vi "NMRController.vi"() -> ()   [LabVIEW 2023]
uses:
  typeDefs/TimeUnits.ctl
  typeDefs/SystemStates.ctl
  <vilib>/DAQmx/write.llb/DAQmx Write (Analog 1D DBL 1Chan NSamp).vi
  <vilib>/DAQmx/read.llb/DAQmx Read (Analog DBL 1Chan 1Samp).vi
  <vilib>/DAQmx/create/channels.llb/DAQmx Create Channel (AI-Voltage-Basic).vi
  <vilib>/DAQmx/configure/timing.llb/DAQmx Timing (Sample Clock).vi
  <vilib>/DAQmx/configure/trigger.llb/DAQmx Start Trigger (Digital Edge).vi
  <vilib>/DAQmx/create/channels.llb/DAQmx Create Channel (AO-Voltage-Basic).vi
  <vilib>/DAQmx/miscellaneous.llb/DAQmx Fill In Error Info.vi
panel:
  in  "STOP":bool
  in  "NMR Signal":tag
  in  "Calibration Antenna":tag
  in  "External Start":tag
  in  "Timed Trigger":bool
  in  "Trigger":bool
  in  "Time Units":T1
  in  "Gathering Time":dbl
  in  "Settings":bool
  out "Voltage Data":dbl[](graph)
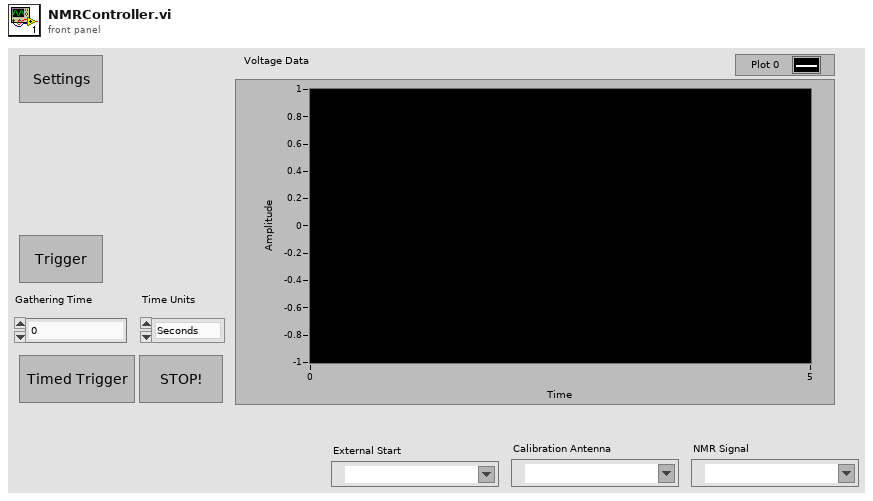
[diagram p1: front panel]
types:
  T1 = typedef "TimeUnits.ctl" = enum16{"Seconds", "Minutes", "Hours"}
  T2 = typedef "SystemStates.ctl" = enum16{"Idle", "Initialize", "Acquire", "Stop", "Shutdown", "Calibrate", "Settings", "I/O"}
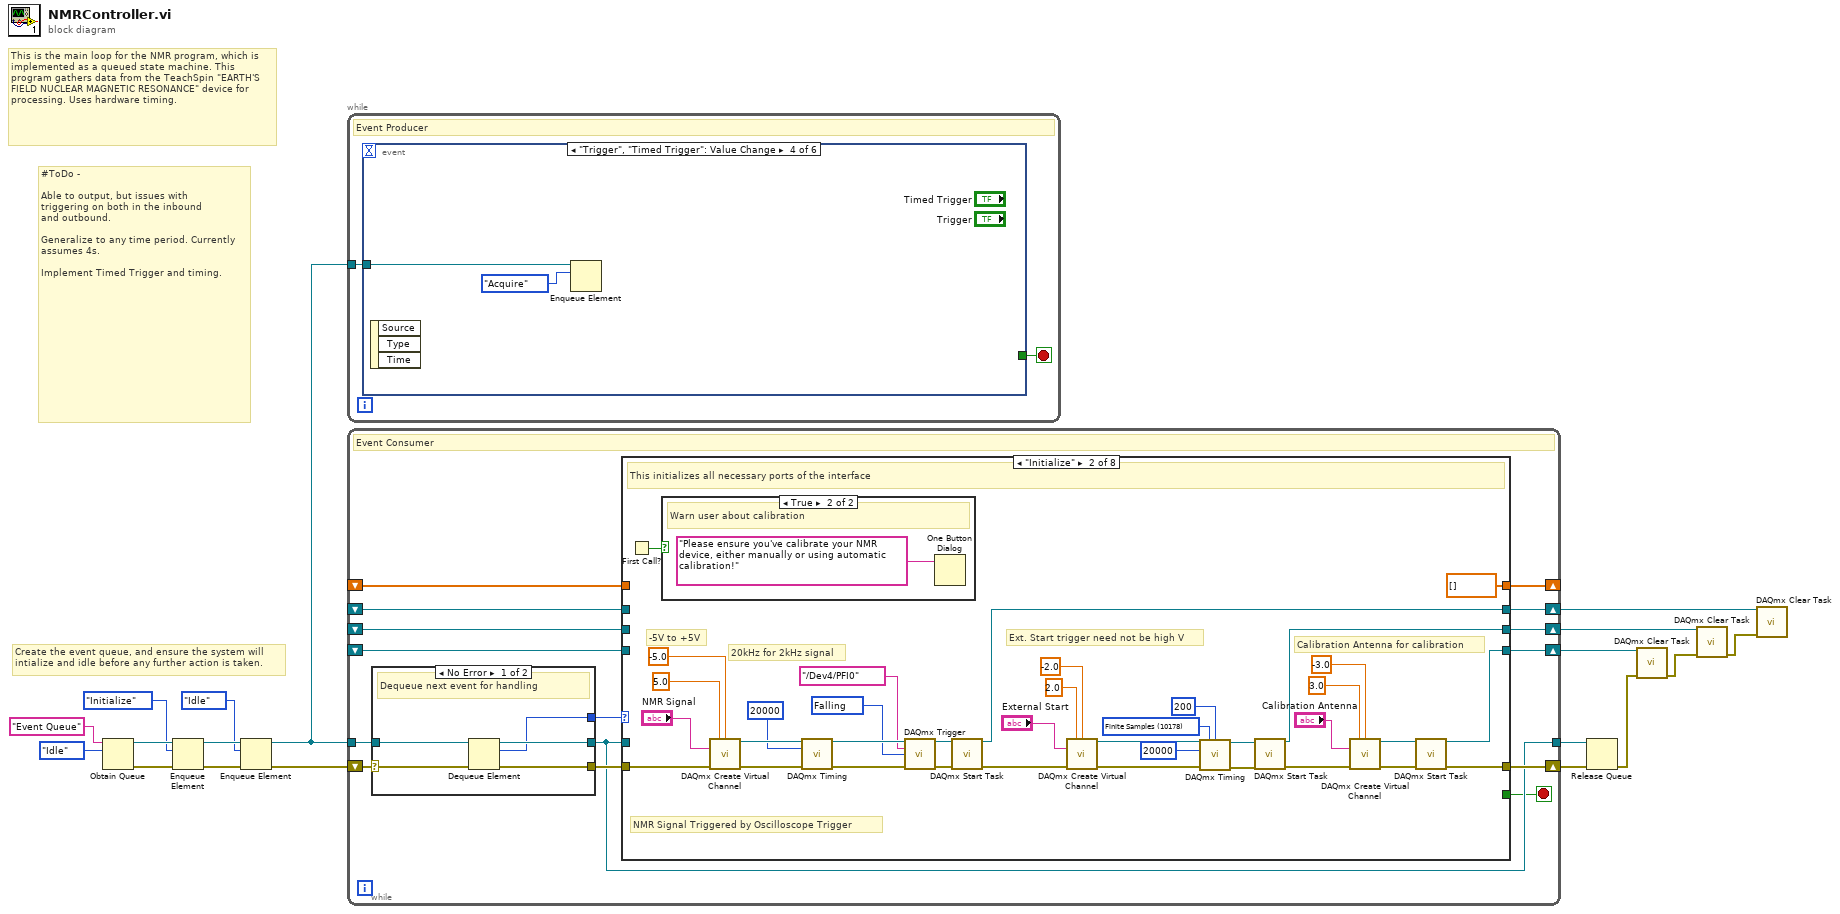
[diagram p0: block diagram]
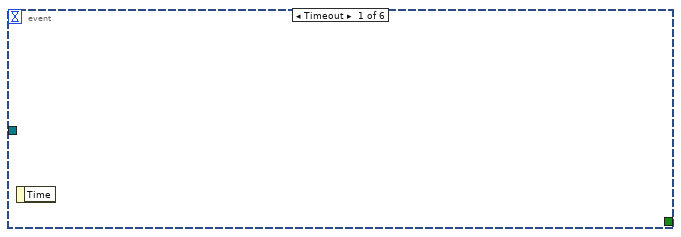
[diagram p2: hidden frame]
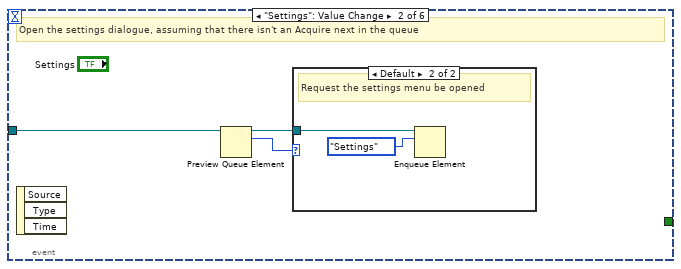
[diagram p3: hidden frame]
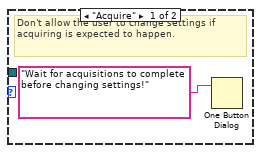
[diagram p4: hidden frame]
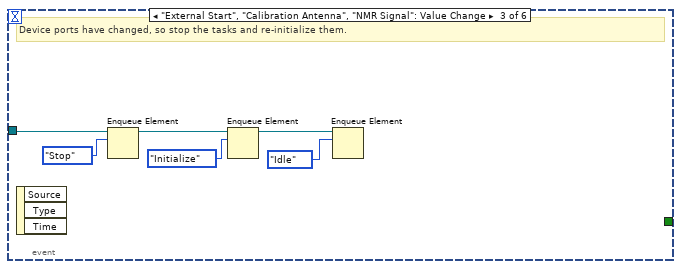
[diagram p5: hidden frame]
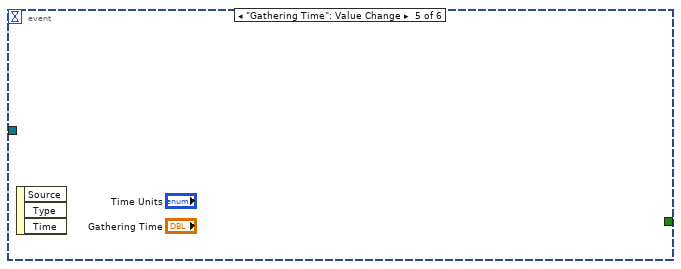
[diagram p6: hidden frame]
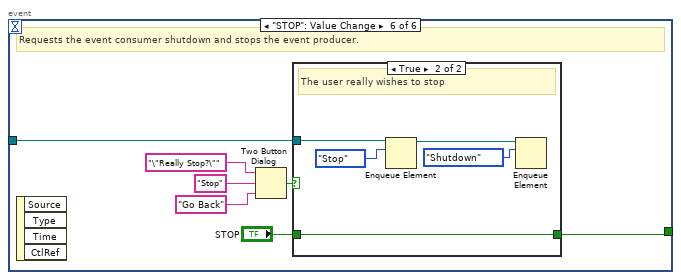
[diagram p7: hidden frame]
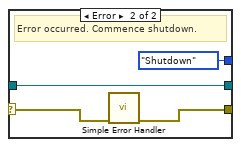
[diagram p9: hidden frame]
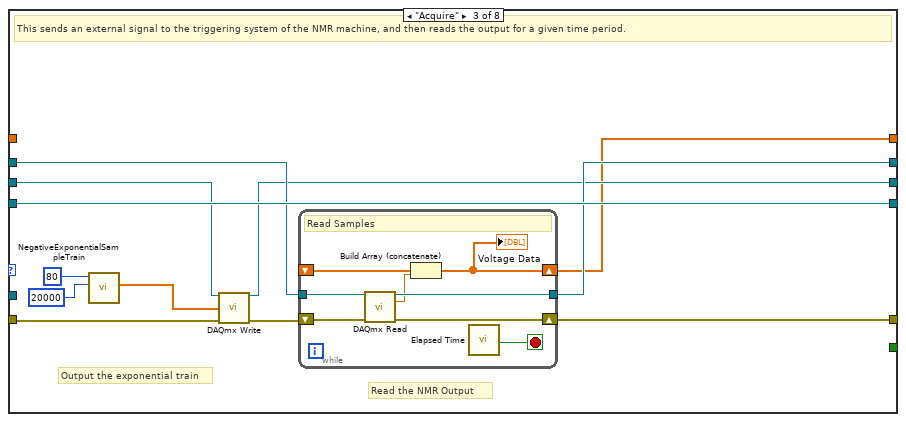
[diagram p12: hidden frame]
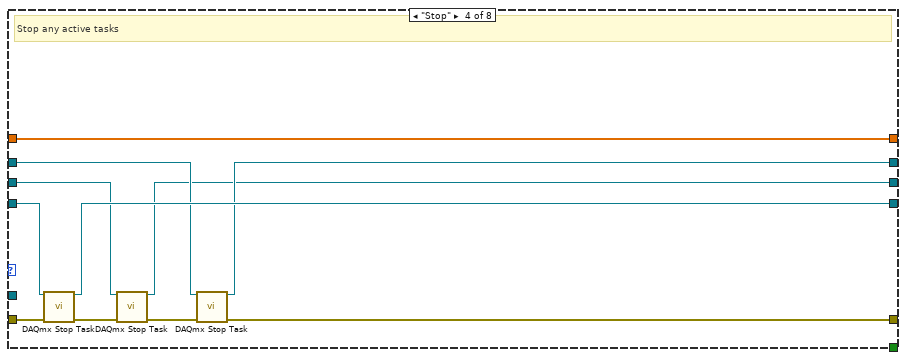
[diagram p13: hidden frame]
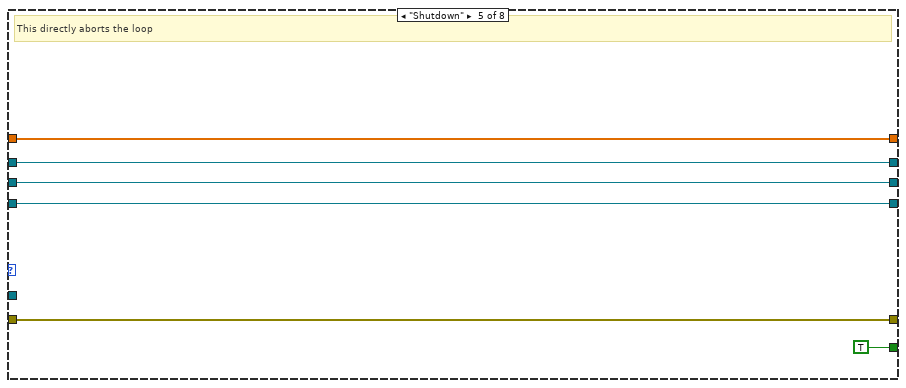
[diagram p14: hidden frame]
diagram:
  # "#ToDo - \n\nAble to output, but issues with\ntriggering on both in the inbound\nand outbound.\n\nGeneralize to any time period. Currently assumes 4s.\n\nImplement Timed Trigger and timing."
  # "This is the main loop for the NMR program, which is implemented as a queued state machine. This program gathers data from the TeachSpin \"EARTH'S FIELD NUCLEAR MAGNETIC RESONANCE\" device for processing. Uses hardware timing."
  # "Create the event queue, and ensure the system will intialize and idle before any further action is taken."
  n1 = Obtain Queue(name (unnamed)="Event Queue", element data type=SystemStates."Idle" ("States")) -> (queue out=w17:refnum<queue>, error out=w13:errorcluster)  [unwired: 3 in, 1 out]
  n2 = Enqueue Element(queue=w17, element=SystemStates."Initialize", error in (no error)=w13) -> (queue out=w16:refnum<queue>, error out=w12:errorcluster)  [unwired: 1 in, 1 out]
  n3 = Enqueue Element(queue=w16, element=SystemStates."Idle", error in (no error)=w12) -> (queue out=w15:refnum<queue>, error out=w14:errorcluster)  [unwired: 1 in, 1 out]
  n4 = while {
    tunnel: w15 -> [w20]
    stop <- w19 stop-if-true
    # "Event Producer"
    n5 = event shown="[3] \"Trigger\", \"Timed Trigger\": Value Change" {
      selector: _ -> [_ _ _ _ _ _]
      dyn-events: _ -> [_ _ _ _ _ _]
      timeout: _ -> [_ _ _ _ _ _]
      tunnel: w20 -> [_ w23 w32 w34 _ w38]
      tunnel: [_ _ _ _ _ w35] -> w19
      event Timeout {
        n6 = event-data() -> ()  [unwired: 1 in, 1 out]
      }
      event "Settings": Value Change {
        # "Open the settings dialogue, assuming that there isn't an Acquire next in the queue"
        n7 = event-data() -> ()  [unwired: 1 in, 3 out]
        n8 = Preview Queue Element(queue=w23) -> (queue out=w21:refnum<queue>, element=w22:T2)  [unwired: 2 in, 2 out]
        n9 = case shown="Default" w22 {
          tunnel: w21 -> [_ w25]
          frame "Acquire" {
            # "Don't allow the user to change settings if acquiring is expected to happen."
            n10 = One Button Dialog(message="Wait for acquisitions to complete before changing settings!") -> ()  [unwired: 1 in, 1 out]
          }
          frame Default {
            # "Request the settings menu be opened"
            n11 = Enqueue Element(queue=w25, element=SystemStates."Settings") -> ()  [unwired: 2 in, 3 out]
          }
        }
      }
      event "External Start", "Calibration Antenna", "NMR Signal": Value Change {
        # "Device ports have changed, so stop the tasks and re-initialize them."
        n12 = event-data() -> ()  [unwired: 1 in, 3 out]
        n13 = Enqueue Element(queue=w32, element=SystemStates."Stop") -> (queue out=w30:refnum<queue>)  [unwired: 2 in, 2 out]
        n14 = Enqueue Element(queue=w30, element=SystemStates."Initialize") -> (queue out=w29:refnum<queue>)  [unwired: 2 in, 2 out]
        n15 = Enqueue Element(queue=w29, element=SystemStates."Idle") -> ()  [unwired: 2 in, 3 out]
      }
      event "Trigger", "Timed Trigger": Value Change {
        n16 = event-data() -> ()  [unwired: 1 in, 3 out]
        n17 = Enqueue Element(queue=w34, element=SystemStates."Acquire") -> ()  [unwired: 2 in, 3 out]
      }
      event "Gathering Time": Value Change {
        n18 = event-data() -> ()  [unwired: 1 in, 3 out]
      }
      event "STOP": Value Change {
        # "Requests the event consumer shutdown and stops the event producer."
        n19 = event-data() -> ()  [unwired: 1 in, 4 out]
        n20 = Two Button Dialog(message="\"Really Stop?\"", 1:"Go Back" ("F button name (\"Cancel\")"), 2:"Stop" ("T button name (\"OK\")")) -> (T button?=w37:bool)
        n21 = case shown="True" w37 {
          tunnel: w38 -> [_ w43]
          tunnel: "STOP" -> [_ w42]
          tunnel: [_ w42] -> w35
          frame False {
            # "The user wants to go back"
          }
          frame True {
            # "The user really wishes to stop"
            n22 = Enqueue Element(queue=w43, element=SystemStates."Stop") -> (queue out=w45:refnum<queue>)  [unwired: 2 in, 2 out]
            n23 = Enqueue Element(queue=w45, element=SystemStates."Shutdown") -> ()  [unwired: 2 in, 3 out]
          }
        }
      }
    }
  }
  n24 = while {
    tunnel: w15 -> [w58]
    shift-right: [w61] -> w7
    shift-left: w14 -> [w59]
    tunnel: [w55] -> w8
    shift-right: [w56] -> w6
    shift-left: _ -> [w53]
    shift-right: [w52] -> w4
    shift-left: _ -> [w51]
    shift-right: [w50] -> w3
    shift-left: _ -> [w49]
    shift-right: [w48] -> _
    shift-left: _ -> [w47]
    stop <- w54 stop-if-true
    # "Event Consumer"
    n25 = case shown="No Error" w59 {
      selector: w59 -> [w66 w68]
      tunnel: [w65 w67] -> w60
      tunnel: w58 -> [w64 w69]
      tunnel: [w63 w69] -> w55
      tunnel: [w62 SystemStates."Shutdown" ("States")] -> w57
      frame No Error {
        # "Dequeue next event for handling"
        n26 = Dequeue Element(queue=w64, error in (no error)=w66) -> (queue out=w63:refnum<queue>, element=w62:T2, error out=w65:errorcluster)  [unwired: 1 in, 1 out]
      }
      frame Error {
        # "Error occurred. Commence shutdown."
        n27 = call <vilib>:"Simple Error Handler.vi"("error in (no error)"=w68) -> ("error out"=w67:errorcluster)  [unwired: 4 in, 4 out]
      }
    }
    n28 = case shown="\"Initialize\"" w57 {
      tunnel: [w75 w91 w123 w141 w149 w154 w159 w164] -> w61
      tunnel: w60 -> [w75 w110 w119 w142 w149 w154 w159 w164]
      tunnel: w55 -> [_ _ _ _ _ _ _ _]
      tunnel: [w74 w90 w124 w140 w147 w153 w158 w163] -> w56
      tunnel: [_ _ _ _ TRUE _ _ _] -> w54
      tunnel: w53 -> [w74 _ w124 w143 w147 w153 w158 w163]
      tunnel: [w73 w98 w121 w138 w146 w152 w157 w162] -> w52
      tunnel: w51 -> [w73 _ w122 w139 w146 w152 w157 w162]
      tunnel: [w72 w88 w114 w134 w145 w151 w156 w161] -> w50
      tunnel: w49 -> [w72 _ w115 w135 w145 w151 w156 w161]
      tunnel: [w71 dbl[] [] w113 w133 w144 w150 w155 w160] -> w48
      tunnel: w47 -> [w71 _ _ w133 w144 w150 w155 w160]
      frame "Idle", Default {
      }
      frame "Initialize" {
        w77 = 10171 items=["Rising"=10280, "Falling"=10171] ("edge")
        w83 = 10178 items=["Finite Samples"=10178, "Continuous Samples"=10123, "Hardware Timed Single Point"=12522] ("sample mode")
        # "Calibration Antenna for calibration"
        # "Ext. Start trigger need not be high V"
        # "NMR Signal Triggered by Oscilloscope Trigger"
        # "-5V to +5V"
        # "20kHz for 2kHz signal"
        # "This initializes all necessary ports of the interface"
        n29 = First Call?() -> (First Call?: T/F=w111:bool)
        n30 = case shown="True" w111 {
          frame False {
            # "Re-initialization, no need to warn the user"
          }
          frame True {
            # "Warn user about calibration"
            n31 = One Button Dialog(message="Please ensure you've calibrate your NMR device, either manually or using automatic calibration!" ("button name (\"OK\")")) -> ()  [unwired: 1 in, 1 out]
          }
        }
        n32 = call-poly <vilib>:"DAQmx Create Virtual Channel.vi"("maximum value"=5.0, "minimum value"=-5.0, "physical channels"="NMR Signal", "error in"=w110) -> ("task out"=w102:refnum<k21>, "error out"=w104:errorcluster)  [unwired: 10 in]
        n33 = call-poly <vilib>:"DAQmx Timing.vi"("task/channels in"=w102, "rate"=20000, "error in"=w104) -> ("task out"=w101:refnum<k21>, "error out"=w103:errorcluster)  [unwired: 11 in]
        n34 = call-poly <vilib>:"DAQmx Trigger.vi"("task/channels in"=w101, "source"=tag "/Dev4/PFI0", "edge"=w77, "error in"=w103) -> ("task out"=w99:refnum<k21>, "error out"=w97:errorcluster)  [unwired: 10 in]
        n35 = call <vilib>:"DAQmx Start Task.vi"("task/channels in"=w99, "error in"=w97) -> ("task out"=w98:refnum<k21>, "error out"=w96:errorcluster)  [unwired: 12 in]
        n36 = call-poly <vilib>:"DAQmx Create Virtual Channel.vi"("maximum value"=2.0, "minimum value"=-2.0, "physical channels"="External Start", "error in"=w96) -> ("task out"=w87:refnum<k21>, "error out"=w86:errorcluster)  [unwired: 10 in]
        n37 = call-poly <vilib>:"DAQmx Timing.vi"("task/channels in"=w87, "sample mode"=w83, "samples per channel"=200, "rate"=20000, "error in"=w86) -> ("task out"=w84:refnum<k21>, "error out"=w85:errorcluster)  [unwired: 9 in]
        n38 = call <vilib>:"DAQmx Start Task.vi"("task/channels in"=w84, "error in"=w85) -> ("task out"=w88:refnum<k21>, "error out"=w93:errorcluster)  [unwired: 12 in]
        n39 = call-poly <vilib>:"DAQmx Create Virtual Channel.vi"("maximum value"=3.0, "minimum value"=-3.0, "physical channels"="Calibration Antenna", "error in"=w93) -> ("task out"=w89:refnum<k21>, "error out"=w92:errorcluster)  [unwired: 10 in]
        n40 = call <vilib>:"DAQmx Start Task.vi"("task/channels in"=w89, "error in"=w92) -> ("task out"=w90:refnum<k21>, "error out"=w91:errorcluster)  [unwired: 12 in]
      }
      frame "Acquire" {
        # "Read the NMR Output"
        # "Output the exponential train"
        # "This sends an external signal to the triggering system of the NMR machine, and then reads the output for a given time period."
        n41 = call "NegativeExponentialSampleTrain.vi"("Sample rate"=20000 ("rate"), "Time (ms)"=80) -> ("ImpulseTrain"=w118:dbl[])  [unwired: 9 in]
        n42 = call-poly <vilib>:"DAQmx Write.vi"("task/channels in"=w115, "data"=w118, "error in"=w119) -> ("task out"=w114:refnum<k21>, "error out"=w120:errorcluster)  [unwired: 10 in, 1 out]
        n43 = while {
          shift-right: [w131] -> w123
          shift-left: w120 -> [w132]
          tunnel: w122 -> [w130]
          tunnel: [w129] -> w121
          shift-right: [w125] -> w113
          shift-left: _ -> [w126]
          stop <- w128 stop-if-true
          # "Read Samples"
          n44 = call-poly <vilib>:"DAQmx Read.vi"("task/channels in"=w130, "error in"=w132) -> ("task out"=w129:refnum<k21>, "data"=w127:dbl, "error out"=w131:errorcluster)  [unwired: 11 in]
          n45 = Build Array (concatenate)(w126, w127) -> (w125:dbl[])
          "Voltage Data" <- w125
          n46 = call "Elapsed Time"() -> ("Time has Elapsed"=w128:bool)  [unwired: 12 in, 7 out]
        }
      }
      frame "Stop" {
        # "Stop any active tasks"
        n47 = call <vilib>:"DAQmx Stop Task.vi"("task/channels in"=w143, "error in"=w142) -> ("task out"=w140:refnum<k21>, "error out"=w137:errorcluster)  [unwired: 12 in]
        n48 = call <vilib>:"DAQmx Stop Task.vi"("task/channels in"=w135, "error in"=w137) -> ("task out"=w134:refnum<k21>, "error out"=w136:errorcluster)  [unwired: 12 in]
        n49 = call <vilib>:"DAQmx Stop Task.vi"("task/channels in"=w139, "error in"=w136) -> ("task out"=w138:refnum<k21>, "error out"=w141:errorcluster)  [unwired: 12 in]
      }
      frame "Shutdown" {
        # "This directly aborts the loop"
      }
      frame "Calibrate" {
        # "TBI: Automated calibration of the system"
      }
      frame "Settings" {
        # "Opens the settings menu"
      }
      frame "I/O" {
        # "I/O setting"
      }
    }
  }
  n50 = Release Queue(queue=w8, error in (no error)=w7) -> (error out=w5:errorcluster)  [unwired: 1 in, 2 out]
  n51 = call <vilib>:"DAQmx Clear Task.vi"("task in"=w6, "error in"=w5) -> ("error out"=w2:errorcluster)  [unwired: 13 in]
  n52 = call <vilib>:"DAQmx Clear Task.vi"("task in"=w3, "error in"=w2) -> ("error out"=w1:errorcluster)  [unwired: 13 in]
  n53 = call <vilib>:"DAQmx Clear Task.vi"("task in"=w4, "error in"=w1) -> ()  [unwired: 13 in, 1 out]
